vi "Lookup Source Groups.vi"(8 "error in (no error)":errorcluster, 11 "ChartGuiTask in":refnum<class "ChartGuiTask.lvclass">) -> (0 "error out":errorcluster, 3 "ChartGuiTask out":refnum<class "ChartGuiTask.lvclass">)   [LabVIEW 2020, in "VolatusDemo.lvlib" / "ChartGuiTask.lvclass"]
uses:
  ChartGuiTask.lvclass
  ChartGuiTask.lvclass/ChartGuiTask.ctl
  Volatus/Task/Task.lvclass
  lv-cdm/CDM-Config/Config Element/Config Element.lvclass
  C:/dev/lv20CE/relink/lv-volatus/Volatus/Task/Task.lvclass
  C:/Program Files (x86)/National Instruments/LabVIEW 2020/vi.lib/ActorFramework/Actor/Actor.lvclass
  C:/dev/lv20CE/relink/lv-volatus/Volatus/TaskStateHandler/TaskStateHandler.lvclass
  C:/dev/lv20CE/relink/lv-volatus/Volatus/VectoMessageHandler/VectoMessageHandler.lvclass
  C:/dev/lv20CE/relink/lv-volatus/VolatusDemo/ChartGuiTask/ChartGuiTask.lvclass
  lv-vecto/Vecto/Group/Group.lvclass
  VolatusConfig/VolatusConfigElement/VolatusConfigElement.lvclass
  VolatusConfig/Task/Task.lvclass
  C:/dev/lv20CE/relink/lv-volatus/VolatusConfig/VolatusConfigElement/VolatusConfigElement.lvclass
  C:/dev/lv20CE/relink/lv-volatus/VolatusConfig/Task/Task.lvclass
  C:/dev/lv20CE/relink/lv-vecto/Vecto/GroupAbstract/GroupAbstract.lvclass
  C:/dev/lv20CE/relink/lv-vecto/Vecto/Group/Group.lvclass
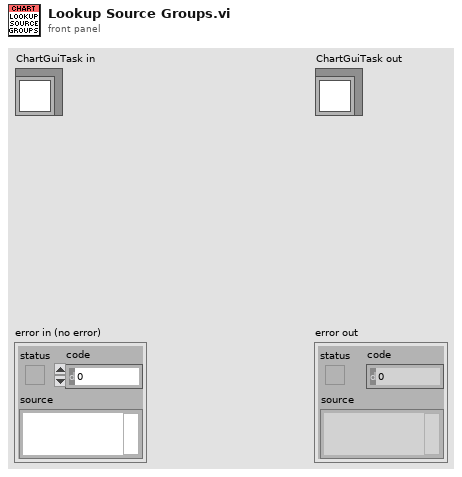
[diagram p1: front panel]
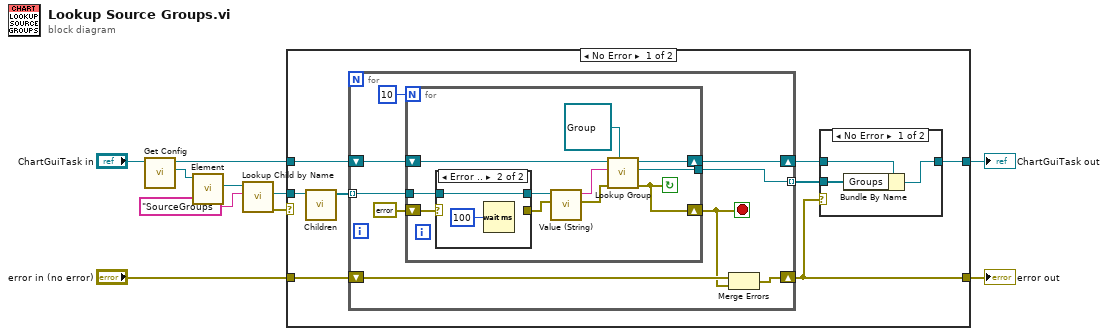
[diagram p0: block diagram]
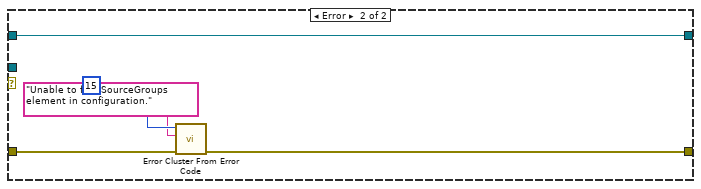
[diagram p4: hidden frame]
diagram:
  n1 = call "Get Config.vi"("Task in"="ChartGuiTask in") -> ("Config"=w10:refnum<class "Task.lvclass">, "Task out"=w4:refnum<class "ChartGuiTask.lvclass">)  [unwired: 8 in, 1 out]
  n2 = call "Element.vi"("VolatusConfigElement in"=w10) -> ("Element"=w8:refnum<class "Config Element.lvclass">)  [unwired: 9 in, 1 out]
  n3 = call "Lookup Child by Name.vi"("Name"="SourceGroups", "Config Element in"=w8) -> ("error out"=w6:errorcluster, "Child"=w5:refnum<class "Config Element.lvclass">)  [unwired: 6 in, 2 out]
  n4 = case shown="No Error" w6 {
    tunnel: w5 -> [w18 _]
    tunnel: w4 -> [w15 w47]
    tunnel: "error in (no error)" -> [w17 w51]
    tunnel: [w13 w48] -> w2
    tunnel: [w12 w47] -> w1
    frame No Error {
      n5 = call "Children.vi"("Config Element in"=w18) -> ("Elements"=w16:refnum<class "Config Element.lvclass">[])  [unwired: 9 in, 1 out]
      n6 = for {
        shift-right: [w28] -> w13
        shift-left: w17 -> [w27]
        tunnel: w16 -> [w31] mode=indexing
        shift-right: [w26] -> w14
        shift-left: w15 -> [w30]
        tunnel: [w29] -> w11 mode=indexing
        stop <- w23 stop-if-true
        n7 = for {
          N: 10 -> [_]
          tunnel: w31 -> [w35]
          tunnel: [w38] -> w29
          shift-right: [w37] -> w26
          shift-left: w30 -> [w42]
          shift-right: [w32] -> w23
          shift-left: errorcluster {"status"=FALSE, "code"=0, "source"=""} ("error out") -> [w36]
          stop <- w32 continue-if-true
          n8 = case shown="Error .." w36 {
            selector: w36 -> [w43 _]
            tunnel: w35 -> [w44 w45]
            tunnel: [w44 w45] -> w34
            tunnel: [w43 _] -> w33
            frame No Error {
            }
            frame Error {
              n9 = Wait (ms)(milliseconds to wait=u32 100) -> ()  [unwired: 1 out]
            }
          }
          n10 = call "Value (String).vi"("error in (no error)"=w33, "Config Element in"=w34) -> ("error out"=w40:errorcluster, "String Value"=w41:string)  [unwired: 8 in]
          n11 = call "Lookup Group.vi"("Group Type (Abstract)"=refnum<class "Group.lvclass"> refnum ("Vecto.lvlib:Group.lvclass"), "error in (no error)"=w40, "Group Name"=w41, "Task in"=w42) -> ("error out"=w32:errorcluster, "Group"=w38:refnum<class "Group.lvclass">, "Task out"=w37:refnum<class "ChartGuiTask.lvclass">)  [unwired: 5 in]
        }
        n12 = Merge Errors(w27, w23) -> (w28:errorcluster)
      }
      n13 = case shown="No Error" w13 {
        tunnel: w14 -> [w21 w22]
        tunnel: [w19 w22] -> w12
        tunnel: w11 -> [w20 _]
        frame No Error {
          n14 = Bundle By Name(cluster=w21, "Groups"=w20) -> (w19:refnum<class "ChartGuiTask.lvclass">)
        }
        frame Error {
        }
      }
    }
    frame Error {
      n15 = call <vilib>:"Error Cluster From Error Code.vi"("error in (no error)"=w51, "error message (\"\")"="Unable to find SourceGroups element in configuration.", "error code (0)"=15) -> ("error out"=w48:errorcluster)  [unwired: 6 in]
    }
  }
  "error out" <- w2
  "ChartGuiTask out" <- w1
